vi "nanocal-frontend-client-LV19.vi"() -> ()   [LabVIEW 2019]
panel:
  out "data":dbl
  out "Numeric":i32
  in  "milliseconds to wait":u32=89
  in  "stop":bool
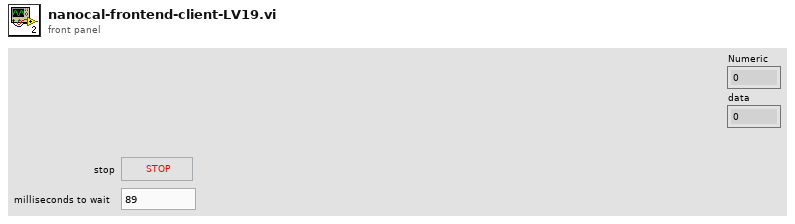
[diagram p1: front panel]
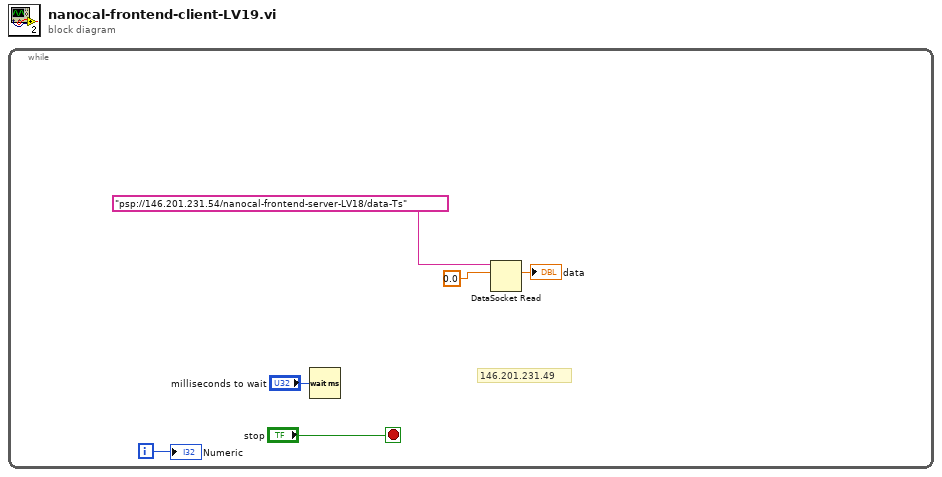
[diagram p0: block diagram]
diagram:
  n1 = while {
    i -> [w4]
    stop <- "stop" stop-if-true
    # "146.201.231.49"
    n2 = Wait (ms)(milliseconds to wait="milliseconds to wait") -> ()  [unwired: 1 out]
    n3 = DataSocket Read(10:0.0, 11:"psp://146.201.231.54/nanocal-frontend-server-LV18/data-Ts" ("connection in")) -> (2:→"data":dbl)  [unwired: 3 in, 6 out]
    "Numeric" <- w4
  }
